vi "unscale lecroy waveform.vi"(11 "Waveform Data":waveform(dbl)[](graph)) -> (2 "GEECS waveforms info":T1(array[cluster]), 3 "scope traces":i16[][](array[numeric]))   [LabVIEW 2013]
uses:
  TektronixDPOSimple.lvclass
panel:
  out "Waveform Data 3":waveform(dbl)[](graph)
  out "Waveform Data 2":waveform(dbl)[](graph)
  out "waveform info out":T2
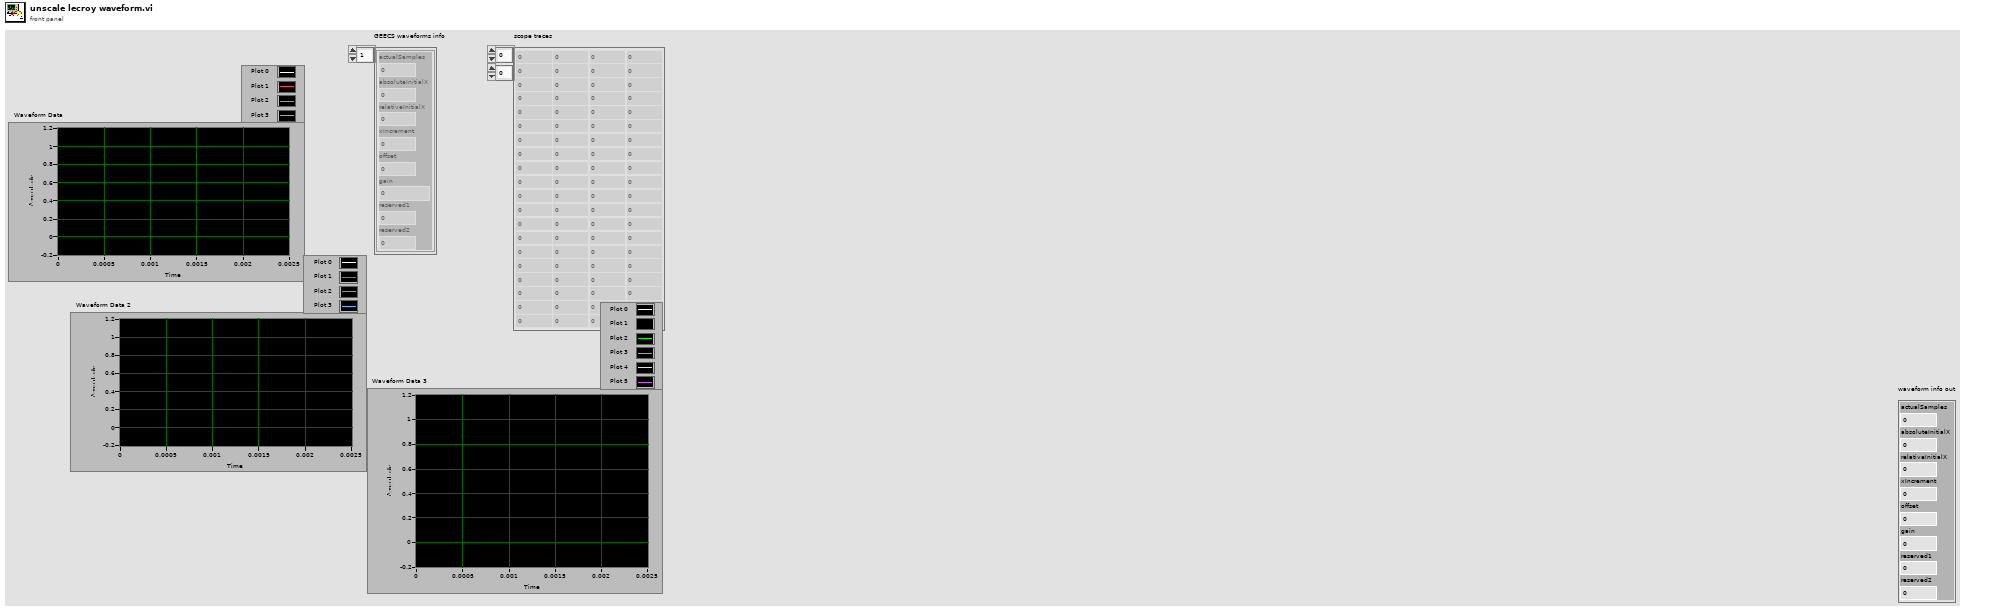
[diagram p1: front panel]
types:
  T1 = cluster{"actualSamples":i32, "absoluteInitialX":dbl, "relativeInitialX":dbl, "xIncrement":dbl, "offset":dbl, "gain":dbl, "reserved1":dbl, "reserved2":dbl}[]
  T2 = cluster{"actualSamples":i32, "absoluteInitialX":dbl, "relativeInitialX":dbl, "xIncrement":dbl, "offset":dbl, "gain":dbl, "reserved1":dbl, "reserved2":dbl}
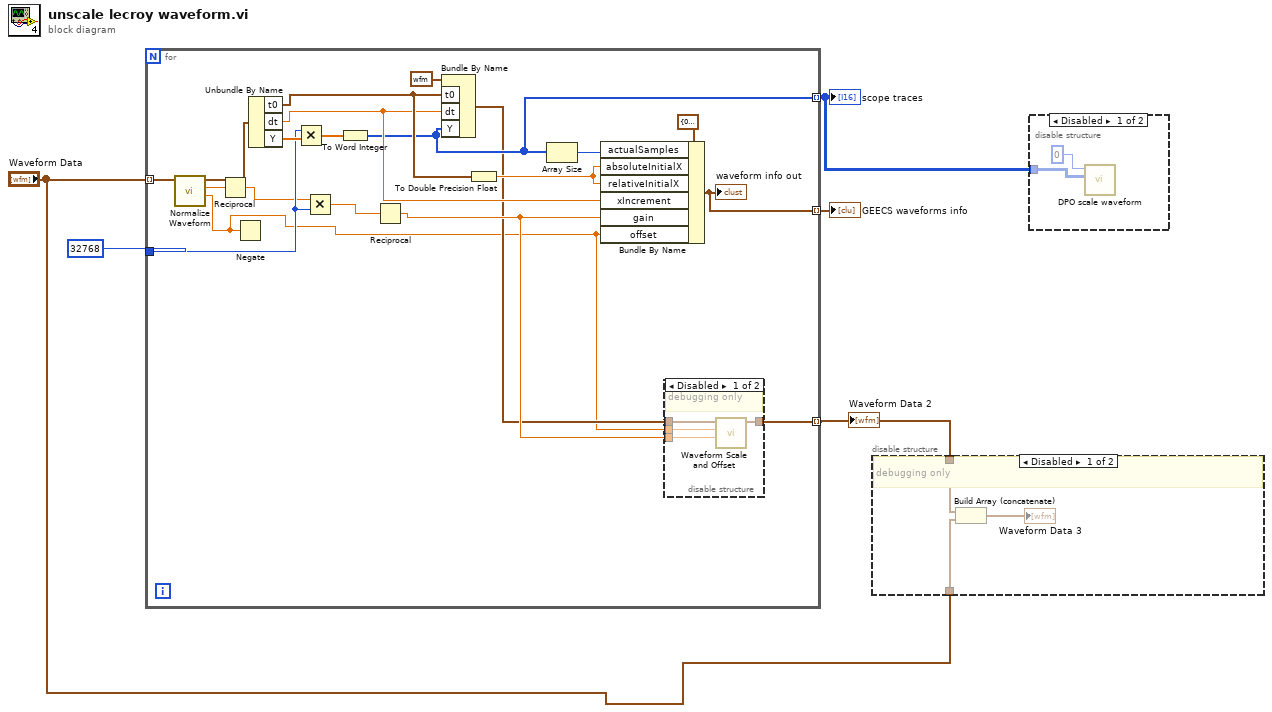
[diagram p0: block diagram]
diagram:
  n1 = for {
    tunnel: "Waveform Data" -> [w21] mode=indexing
    tunnel: 32768 -> [w23]
    tunnel: [w17] -> w3 mode=indexing
    tunnel: [w13] -> w4 mode=indexing
    tunnel: [w9] -> w2 mode=indexing
    n2 = call "Normalize Waveform.vi"("waveform in"=w21) -> ("offset"=w6:dbl, "scale"=w8:dbl, "normalized waveform"=w25:waveform(dbl))  [unwired: 7 in, 1 out]
    n3 = Reciprocal(x=w8) -> (1/x=w7:dbl)
    n4 = Negate(x=w6) -> ()  [unwired: 1 out]
    n5 = Unbundle By Name(w25) -> ("t0"=w15:timestamp, "dt"=w14:dbl, "Y"=w24:dbl[])
    n6 = Multiply(x=w23, y=w24) -> (x*y=w22:dbl[])
    n7 = Multiply(x=w7, y=w23) -> (x*y=w12:dbl)
    n8 = To Word Integer(number=w22) -> (16bit integer=w13:i16[])
    n9 = Reciprocal(x=w12) -> (1/x=w11:dbl)
    n10 = Bundle By Name(cluster=waveform(i16) {"t0"=timestamp(0 s since 1904-01-01), "dt"=1.0, "Y"=[]} ("waveform"), "t0"=w15, "dt"=w14, "Y"=w13) -> (w10:waveform(i16))
    n11 = To Double Precision Float(number=w15) -> (double precision float=w16:dbl)
    n12 = Array Size(array=w13) -> (size(s)=w18:i32)
    n13 = Bundle By Name(cluster=T2 {"actualSamples"=0, "absoluteInitialX"=0.0, "relativeInitialX"=0.0, "xIncrement"=0.0, "offset"=0.0, "gain"=0.0, "reserved1"=0.0, "reserved2"=0.0} ("waveform info"), "actualSamples"=w18, "absoluteInitialX"=w16, "relativeInitialX"=w16, "xIncrement"=w14, "gain"=w11, "offset"=w6) -> (w17:T2)
    "waveform info out" <- w17
    n14 = disable-structure shown="Disabled" {
      disable-tunnel: w11 -> [w29 _]
      disable-tunnel: w10 -> [w28 _]
      disable-tunnel: [w27 _] -> w9
      disable-tunnel: w6 -> [w26 _]
      frame Disabled {
        # "debugging only"
        n15 = call "Waveform Scale and Offset.vi"("scale"=w29, "offset"=w26, "waveform in"=w28) -> ("waveform out"=w27:waveform(dbl))  [unwired: 7 in, 1 out]
      }
      frame Enabled {
      }
    }
  }
  "GEECS waveforms info" <- w3
  "scope traces" <- w4
  "Waveform Data 2" <- w2
  n16 = disable-structure shown="Disabled" {
    disable-tunnel: w2 -> [w32 _]
    disable-tunnel: "Waveform Data" -> [w30 _]
    frame Disabled {
      # "debugging only"
      n17 = Build Array (concatenate)(w32, w30) -> (→"Waveform Data 3":waveform(dbl)[])
    }
    frame Enabled {
    }
  }
  n18 = disable-structure shown="Disabled" {
    disable-tunnel: w4 -> [w33 _]
    frame Disabled {
      n19 = call "DPO scale waveform.vi"("I16 in"=w33, "Number of waveforms"=0) -> ()  [unwired: 6 in, 4 out]
    }
    frame Enabled {
    }
  }
